vi "D2SParser - Private - Function - Read Character Stats.vi"(8 "error in (no error)":errorcluster, 11 "D2SParser in":refnum<class "D2SParser.lvclass">) -> (0 "error out":errorcluster, 3 "D2SParser out":refnum<class "D2SParser.lvclass">)   [LabVIEW 2015, in "D2SParser.lvclass"]
uses:
  D2SParser.lvclass
  D2SParser.lvclass/D2SParser.ctl
  D2Character/D2Character.lvclass/D2Character.ctl
  D2Character/D2Character - Accessors - Set Strength.vi
  D2Character/D2Character - Accessors - Set Energy.vi
  D2Character/D2Character - Accessors - Set Dexterity.vi
  D2Character/D2Character - Accessors - Set Vitality.vi
  D2Character/D2Character - Accessors - Set Stat Points Remaining.vi
  D2Character/D2Character - Accessors - Set Skill Points Remaining.vi
  D2Character/D2Character - Accessors - Set Current Life.vi
  D2Character/D2Character - Accessors - Set Life Base.vi
  D2Character/D2Character - Accessors - Set Current Mana.vi
  D2Character/D2Character - Accessors - Set Mana Base.vi
  D2Character/D2Character - Accessors - Set Current Stamina.vi
  D2Character/D2Character - Accessors - Set Stamina Base.vi
  D2Character/D2Character - Accessors - Set Level.vi
  D2Character/D2Character - Accessors - Set Experience.vi
  D2Character/D2Character - Accessors - Set Gold Inventory.vi
  D2Character/D2Character - Accessors - Set Stash Gold.vi
  D2Character/D2Character.lvclass
panel:
  out "ASCII":string
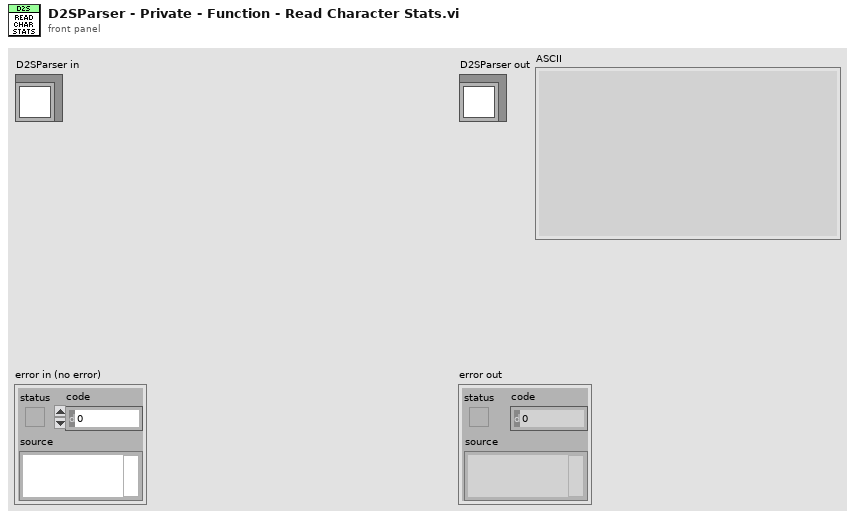
[diagram p1: front panel]
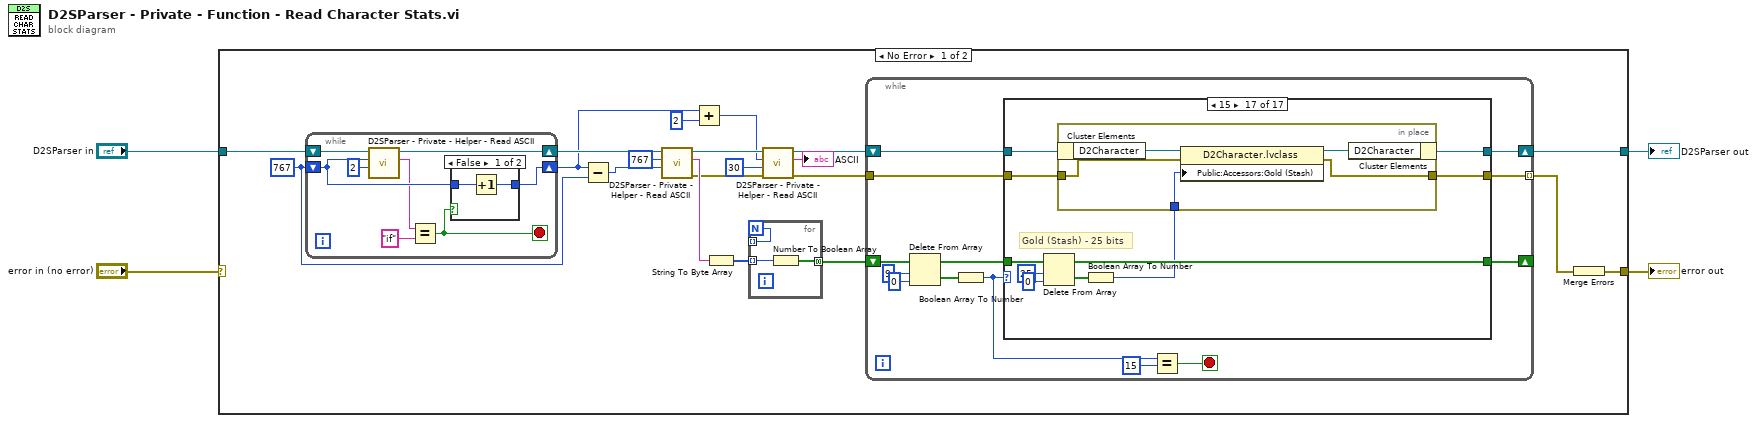
[diagram p0: block diagram]
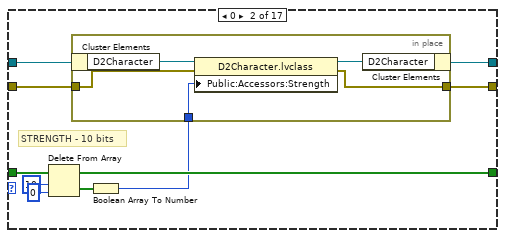
[diagram p3: hidden frame]
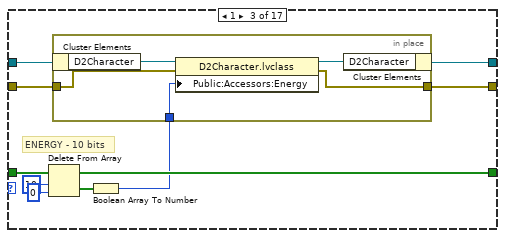
[diagram p4: hidden frame]
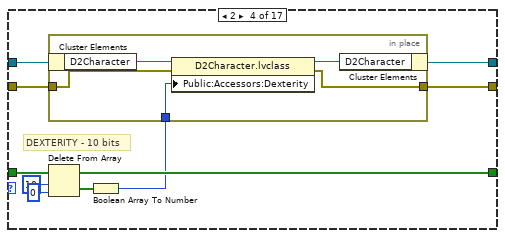
[diagram p5: hidden frame]
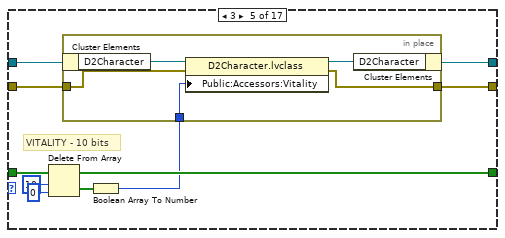
[diagram p6: hidden frame]
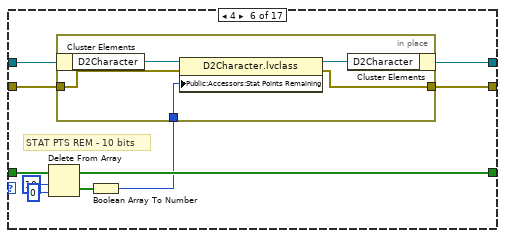
[diagram p7: hidden frame]
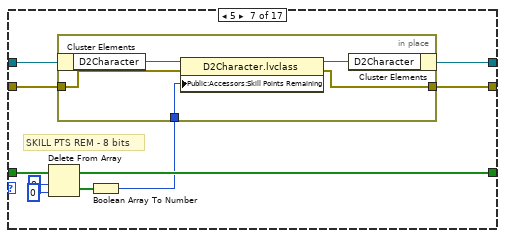
[diagram p8: hidden frame]
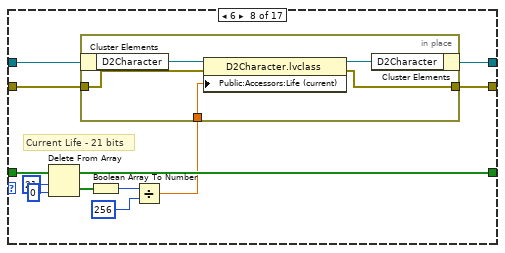
[diagram p9: hidden frame]
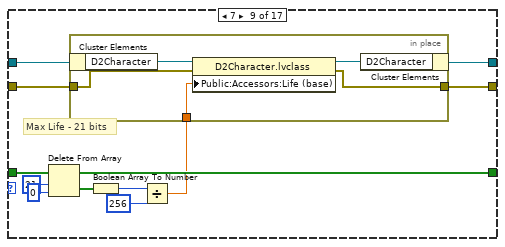
[diagram p10: hidden frame]
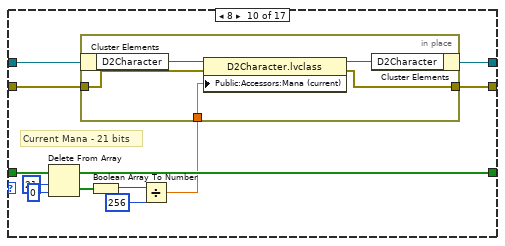
[diagram p11: hidden frame]
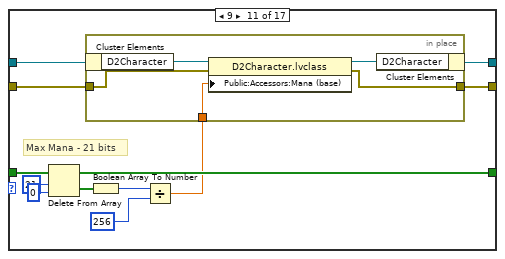
[diagram p12: hidden frame]
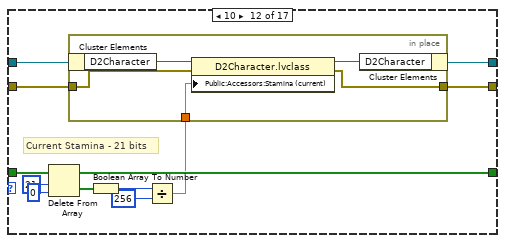
[diagram p13: hidden frame]
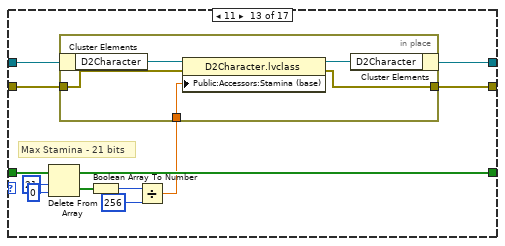
[diagram p14: hidden frame]
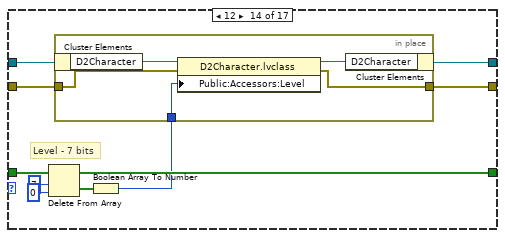
[diagram p15: hidden frame]
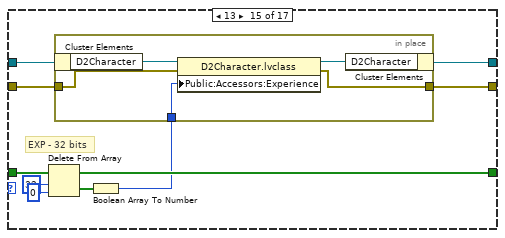
[diagram p16: hidden frame]
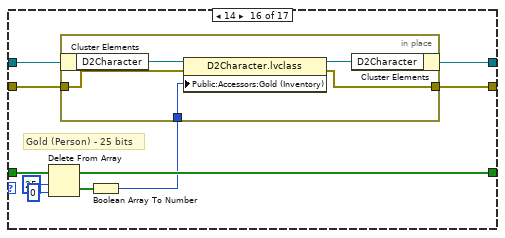
[diagram p17: hidden frame]
diagram:
  n1 = case shown="No Error" "error in (no error)" {
    selector: "error in (no error)" -> [_ w308]
    tunnel: [w22 w308] -> w3
    tunnel: [w23 w307] -> w1
    tunnel: "D2SParser in" -> [w24 w307]
    frame No Error {
      w21 = i64 767 ("Position")
      n2 = while {
        shift-right: [w301] -> w9
        shift-left: w21 -> [w302]
        shift-right: [w296] -> w20
        shift-left: w24 -> [w303]
        stop <- w297 stop-if-true
        n3 = call "D2SParser - Private - Helper - Read ASCII.vi"("# Characters"=2, "Position"=w302, "D2SParser in"=w303) -> ("ASCII"=w299:string, "D2SParser out"=w296:refnum<class "D2SParser.lvclass">)  [unwired: 6 in, 1 out]
        n4 = Equal?(x=w299, y="if") -> (x = y?=w297:bool)
        n5 = case shown="False" w297 {
          tunnel: w302 -> [w305 w306]
          tunnel: [w304 w306] -> w301
          frame False {
            n6 = Increment(x=w305) -> (x+1=w304:i64)
          }
          frame True {
          }
        }
      }
      n7 = Subtract(x=w9, y=w21) -> (x-y=w19:i64)
      n8 = call "D2SParser - Private - Helper - Read ASCII.vi"("# Characters"=w19, "Position"=i64 767, "D2SParser in"=w20) -> ("error out"=w11:errorcluster, "ASCII"=w17:string, "D2SParser out"=w13:refnum<class "D2SParser.lvclass">)  [unwired: 6 in]
      n9 = Add(x=w9, y=i64 2) -> (x+y=w8:i64)
      n10 = String To Byte Array(string=w17) -> (unsigned byte array=w16:u8[])
      n11 = for {
        N -> [w293]
        tunnel: w16 -> [w295] mode=indexing
        tunnel: [w294] -> w15 mode=concatenating
        tunnel: [w293] -> _ mode=indexing
        n12 = Number To Boolean Array(number=w295) -> (Boolean array=w294:bool[])
      }
      n13 = call "D2SParser - Private - Helper - Read ASCII.vi"("error in (no error)"=w11, "# Characters"=i64 30 ("x+y"), "Position"=w8, "D2SParser in"=w13) -> ("error out"=w10:errorcluster, "ASCII"=→"ASCII":string, "D2SParser out"=w12:refnum<class "D2SParser.lvclass">)  [unwired: 5 in]
      n14 = while {
        shift-right: [w32] -> _
        shift-left: w15 -> [w37]
        tunnel: w10 -> [w26]
        tunnel: [w25] -> w14 mode=indexing
        shift-right: [w27] -> w23
        shift-left: w12 -> [w28]
        stop <- w31 stop-if-true
        n15 = Delete From Array(array=w37, length=9, index=0) -> (deleted portion=w34:bool[], array with subset deleted=w33:bool[])
        n16 = Boolean Array To Number(Boolean array=w34) -> (number=w30:u32)
        n17 = case shown="15" w30 {
          tunnel: w33 -> [w40 w50 w65 w80 w95 w110 w125 w142 w159 w176 w193 w210 w227 w242 w257 w272 w287]
          tunnel: [w40 w47 w62 w77 w92 w107 w122 w139 w156 w173 w190 w207 w224 w239 w254 w269 w284] -> w32
          tunnel: w28 -> [w39 w45 w60 w75 w90 w105 w120 w133 w152 w171 w187 w205 w222 w237 w252 w267 w282]
          tunnel: [w39 w43 w57 w72 w88 w103 w118 w132 w149 w166 w186 w203 w220 w234 w249 w265 w279] -> w27
          tunnel: w26 -> [w38 w42 w58 w74 w89 w104 w119 w134 w151 w170 w188 w204 w221 w236 w251 w266 w281]
          tunnel: [w38 w44 w56 w71 w87 w102 w117 w135 w148 w165 w185 w202 w219 w233 w248 w264 w278] -> w25
          frame Default {
          }
          frame 0 {
            # "STRENGTH - 10 bits"
            n18 = Delete From Array(array=w50, length=10, index=0) -> (deleted portion=w46:bool[], array with subset deleted=w47:bool[])
            n19 = Boolean Array To Number(Boolean array=w46) -> (number=w41:u32)
            n20 = in-place {
              in-place-border: [w53] -> w44
              in-place-border: w42 -> [w52]
              in-place-border: w41 -> [w51]
              n21 = in-place-cluster #1(w45) -> ("D2Character"=w55:refnum<class "D2Character.lvclass">)
              n22 = property class="D2Character.lvclass"(reference=w55, error in=w52, "Public:Accessors:Strength"=w51) -> (reference out=w54:refnum<class "D2Character.lvclass">, error out=w53:errorcluster)
              n23 = in-place-cluster #1("D2Character"=w54) -> (w43:refnum<class "D2SParser.lvclass">)
            }
          }
          frame 1 {
            # "ENERGY - 10 bits"
            n24 = Delete From Array(array=w65, length=10, index=0) -> (deleted portion=w61:bool[], array with subset deleted=w62:bool[])
            n25 = Boolean Array To Number(Boolean array=w61) -> (number=w59:u32)
            n26 = in-place {
              in-place-border: [w68] -> w56
              in-place-border: w58 -> [w67]
              in-place-border: w59 -> [w66]
              n27 = in-place-cluster #2(w60) -> ("D2Character"=w70:refnum<class "D2Character.lvclass">)
              n28 = property class="D2Character.lvclass"(reference=w70, error in=w67, "Public:Accessors:Energy"=w66) -> (reference out=w69:refnum<class "D2Character.lvclass">, error out=w68:errorcluster)
              n29 = in-place-cluster #2("D2Character"=w69) -> (w57:refnum<class "D2SParser.lvclass">)
            }
          }
          frame 2 {
            # "DEXTERITY - 10 bits"
            n30 = Delete From Array(array=w80, length=10, index=0) -> (deleted portion=w76:bool[], array with subset deleted=w77:bool[])
            n31 = Boolean Array To Number(Boolean array=w76) -> (number=w73:u32)
            n32 = in-place {
              in-place-border: [w83] -> w71
              in-place-border: w74 -> [w82]
              in-place-border: w73 -> [w81]
              n33 = in-place-cluster #3(w75) -> ("D2Character"=w85:refnum<class "D2Character.lvclass">)
              n34 = property class="D2Character.lvclass"(reference=w85, error in=w82, "Public:Accessors:Dexterity"=w81) -> (reference out=w84:refnum<class "D2Character.lvclass">, error out=w83:errorcluster)
              n35 = in-place-cluster #3("D2Character"=w84) -> (w72:refnum<class "D2SParser.lvclass">)
            }
          }
          frame 3 {
            # "VITALITY - 10 bits"
            n36 = Delete From Array(array=w95, length=10, index=0) -> (deleted portion=w91:bool[], array with subset deleted=w92:bool[])
            n37 = Boolean Array To Number(Boolean array=w91) -> (number=w86:u32)
            n38 = in-place {
              in-place-border: [w98] -> w87
              in-place-border: w89 -> [w97]
              in-place-border: w86 -> [w96]
              n39 = in-place-cluster #4(w90) -> ("D2Character"=w100:refnum<class "D2Character.lvclass">)
              n40 = property class="D2Character.lvclass"(reference=w100, error in=w97, "Public:Accessors:Vitality"=w96) -> (reference out=w99:refnum<class "D2Character.lvclass">, error out=w98:errorcluster)
              n41 = in-place-cluster #4("D2Character"=w99) -> (w88:refnum<class "D2SParser.lvclass">)
            }
          }
          frame 4 {
            # "STAT PTS REM - 10 bits"
            n42 = Delete From Array(array=w110, length=10, index=0) -> (deleted portion=w106:bool[], array with subset deleted=w107:bool[])
            n43 = Boolean Array To Number(Boolean array=w106) -> (number=w101:u32)
            n44 = in-place {
              in-place-border: [w113] -> w102
              in-place-border: w104 -> [w112]
              in-place-border: w101 -> [w111]
              n45 = in-place-cluster #5(w105) -> ("D2Character"=w115:refnum<class "D2Character.lvclass">)
              n46 = property class="D2Character.lvclass"(reference=w115, error in=w112, "Public:Accessors:Stat Points Remaining"=w111) -> (reference out=w114:refnum<class "D2Character.lvclass">, error out=w113:errorcluster)
              n47 = in-place-cluster #5("D2Character"=w114) -> (w103:refnum<class "D2SParser.lvclass">)
            }
          }
          frame 5 {
            # "SKILL PTS REM - 8 bits"
            n48 = Delete From Array(array=w125, length=8, index=0) -> (deleted portion=w121:bool[], array with subset deleted=w122:bool[])
            n49 = Boolean Array To Number(Boolean array=w121) -> (number=w116:u32)
            n50 = in-place {
              in-place-border: [w128] -> w117
              in-place-border: w119 -> [w127]
              in-place-border: w116 -> [w126]
              n51 = in-place-cluster #6(w120) -> ("D2Character"=w130:refnum<class "D2Character.lvclass">)
              n52 = property class="D2Character.lvclass"(reference=w130, error in=w127, "Public:Accessors:Skill Points Remaining"=w126) -> (reference out=w129:refnum<class "D2Character.lvclass">, error out=w128:errorcluster)
              n53 = in-place-cluster #6("D2Character"=w129) -> (w118:refnum<class "D2SParser.lvclass">)
            }
          }
          frame 6 {
            # "Current Life - 21 bits"
            n54 = Delete From Array(array=w142, length=21, index=0) -> (deleted portion=w138:bool[], array with subset deleted=w139:bool[])
            n55 = Boolean Array To Number(Boolean array=w138) -> (number=w137:u32)
            n56 = Divide(x=w137, y=u32 256) -> (x/y=w131:dbl)
            n57 = in-place {
              in-place-border: [w146] -> w135
              in-place-border: w134 -> [w145]
              in-place-border: w131 -> [w144]
              n58 = in-place-cluster #7(w133) -> ("D2Character"=w143:refnum<class "D2Character.lvclass">)
              n59 = property class="D2Character.lvclass"(reference=w143, error in=w145, "Public:Accessors:Life (current)"=w144) -> (reference out=w147:refnum<class "D2Character.lvclass">, error out=w146:errorcluster)
              n60 = in-place-cluster #7("D2Character"=w147) -> (w132:refnum<class "D2SParser.lvclass">)
            }
          }
          frame 7 {
            # "Max Life - 21 bits"
            n61 = Delete From Array(array=w159, length=21, index=0) -> (deleted portion=w155:bool[], array with subset deleted=w156:bool[])
            n62 = Boolean Array To Number(Boolean array=w155) -> (number=w154:u32)
            n63 = Divide(x=w154, y=u32 256) -> (x/y=w150:dbl)
            n64 = in-place {
              in-place-border: [w162] -> w148
              in-place-border: w151 -> [w161]
              in-place-border: w150 -> [w160]
              n65 = in-place-cluster #8(w152) -> ("D2Character"=w164:refnum<class "D2Character.lvclass">)
              n66 = property class="D2Character.lvclass"(reference=w164, error in=w161, "Public:Accessors:Life (base)"=w160) -> (reference out=w163:refnum<class "D2Character.lvclass">, error out=w162:errorcluster)
              n67 = in-place-cluster #8("D2Character"=w163) -> (w149:refnum<class "D2SParser.lvclass">)
            }
          }
          frame 8 {
            # "Current Mana - 21 bits"
            n68 = Delete From Array(array=w176, length=21, index=0) -> (deleted portion=w172:bool[], array with subset deleted=w173:bool[])
            n69 = Boolean Array To Number(Boolean array=w172) -> (number=w169:u32)
            n70 = Divide(x=w169, y=u32 256) -> (x/y=w167:dbl)
            n71 = in-place {
              in-place-border: [w179] -> w165
              in-place-border: w170 -> [w178]
              in-place-border: w167 -> [w177]
              n72 = in-place-cluster #9(w171) -> ("D2Character"=w181:refnum<class "D2Character.lvclass">)
              n73 = property class="D2Character.lvclass"(reference=w181, error in=w178, "Public:Accessors:Mana (current)"=w177) -> (reference out=w180:refnum<class "D2Character.lvclass">, error out=w179:errorcluster)
              n74 = in-place-cluster #9("D2Character"=w180) -> (w166:refnum<class "D2SParser.lvclass">)
            }
          }
          frame 9 {
            # "Max Mana - 21 bits"
            n75 = Delete From Array(array=w193, length=21, index=0) -> (deleted portion=w189:bool[], array with subset deleted=w190:bool[])
            n76 = Boolean Array To Number(Boolean array=w189) -> (number=w184:u32)
            n77 = Divide(x=w184, y=u32 256) -> (x/y=w183:dbl)
            n78 = in-place {
              in-place-border: [w196] -> w185
              in-place-border: w188 -> [w195]
              in-place-border: w183 -> [w194]
              n79 = in-place-cluster #10(w187) -> ("D2Character"=w198:refnum<class "D2Character.lvclass">)
              n80 = property class="D2Character.lvclass"(reference=w198, error in=w195, "Public:Accessors:Mana (base)"=w194) -> (reference out=w197:refnum<class "D2Character.lvclass">, error out=w196:errorcluster)
              n81 = in-place-cluster #10("D2Character"=w197) -> (w186:refnum<class "D2SParser.lvclass">)
            }
          }
          frame 10 {
            # "Current Stamina - 21 bits"
            n82 = Delete From Array(array=w210, length=21, index=0) -> (deleted portion=w206:bool[], array with subset deleted=w207:bool[])
            n83 = Boolean Array To Number(Boolean array=w206) -> (number=w201:u32)
            n84 = Divide(x=w201, y=u32 256) -> (x/y=w199:dbl)
            n85 = in-place {
              in-place-border: [w213] -> w202
              in-place-border: w204 -> [w212]
              in-place-border: w199 -> [w211]
              n86 = in-place-cluster #11(w205) -> ("D2Character"=w215:refnum<class "D2Character.lvclass">)
              n87 = property class="D2Character.lvclass"(reference=w215, error in=w212, "Public:Accessors:Stamina (current)"=w211) -> (reference out=w214:refnum<class "D2Character.lvclass">, error out=w213:errorcluster)
              n88 = in-place-cluster #11("D2Character"=w214) -> (w203:refnum<class "D2SParser.lvclass">)
            }
          }
          frame 11 {
            # "Max Stamina - 21 bits"
            n89 = Delete From Array(array=w227, length=21, index=0) -> (deleted portion=w223:bool[], array with subset deleted=w224:bool[])
            n90 = Boolean Array To Number(Boolean array=w223) -> (number=w218:u32)
            n91 = Divide(x=w218, y=u32 256) -> (x/y=w216:dbl)
            n92 = in-place {
              in-place-border: [w230] -> w219
              in-place-border: w221 -> [w229]
              in-place-border: w216 -> [w228]
              n93 = in-place-cluster #12(w222) -> ("D2Character"=w232:refnum<class "D2Character.lvclass">)
              n94 = property class="D2Character.lvclass"(reference=w232, error in=w229, "Public:Accessors:Stamina (base)"=w228) -> (reference out=w231:refnum<class "D2Character.lvclass">, error out=w230:errorcluster)
              n95 = in-place-cluster #12("D2Character"=w231) -> (w220:refnum<class "D2SParser.lvclass">)
            }
          }
          frame 12 {
            # "Level - 7 bits"
            n96 = Delete From Array(array=w242, length=7, index=0) -> (deleted portion=w238:bool[], array with subset deleted=w239:bool[])
            n97 = Boolean Array To Number(Boolean array=w238) -> (number=w235:u32)
            n98 = in-place {
              in-place-border: [w245] -> w233
              in-place-border: w236 -> [w244]
              in-place-border: w235 -> [w243]
              n99 = in-place-cluster #13(w237) -> ("D2Character"=w247:refnum<class "D2Character.lvclass">)
              n100 = property class="D2Character.lvclass"(reference=w247, error in=w244, "Public:Accessors:Level"=w243) -> (reference out=w246:refnum<class "D2Character.lvclass">, error out=w245:errorcluster)
              n101 = in-place-cluster #13("D2Character"=w246) -> (w234:refnum<class "D2SParser.lvclass">)
            }
          }
          frame 13 {
            # "EXP - 32 bits"
            n102 = Delete From Array(array=w257, length=32, index=0) -> (deleted portion=w253:bool[], array with subset deleted=w254:bool[])
            n103 = Boolean Array To Number(Boolean array=w253) -> (number=w250:u32)
            n104 = in-place {
              in-place-border: [w260] -> w248
              in-place-border: w251 -> [w259]
              in-place-border: w250 -> [w258]
              n105 = in-place-cluster #14(w252) -> ("D2Character"=w262:refnum<class "D2Character.lvclass">)
              n106 = property class="D2Character.lvclass"(reference=w262, error in=w259, "Public:Accessors:Experience"=w258) -> (reference out=w261:refnum<class "D2Character.lvclass">, error out=w260:errorcluster)
              n107 = in-place-cluster #14("D2Character"=w261) -> (w249:refnum<class "D2SParser.lvclass">)
            }
          }
          frame 14 {
            # "Gold (Person) - 25 bits"
            n108 = Delete From Array(array=w272, length=25, index=0) -> (deleted portion=w268:bool[], array with subset deleted=w269:bool[])
            n109 = Boolean Array To Number(Boolean array=w268) -> (number=w263:u32)
            n110 = in-place {
              in-place-border: [w275] -> w264
              in-place-border: w266 -> [w274]
              in-place-border: w263 -> [w273]
              n111 = in-place-cluster #15(w267) -> ("D2Character"=w277:refnum<class "D2Character.lvclass">)
              n112 = property class="D2Character.lvclass"(reference=w277, error in=w274, "Public:Accessors:Gold (Inventory)"=w273) -> (reference out=w276:refnum<class "D2Character.lvclass">, error out=w275:errorcluster)
              n113 = in-place-cluster #15("D2Character"=w276) -> (w265:refnum<class "D2SParser.lvclass">)
            }
          }
          frame 15 {
            # "Gold (Stash) - 25 bits"
            n114 = Delete From Array(array=w287, length=25, index=0) -> (deleted portion=w283:bool[], array with subset deleted=w284:bool[])
            n115 = Boolean Array To Number(Boolean array=w283) -> (number=w280:u32)
            n116 = in-place {
              in-place-border: [w290] -> w278
              in-place-border: w281 -> [w289]
              in-place-border: w280 -> [w288]
              n117 = in-place-cluster #16(w282) -> ("D2Character"=w292:refnum<class "D2Character.lvclass">)
              n118 = property class="D2Character.lvclass"(reference=w292, error in=w289, "Public:Accessors:Gold (Stash)"=w288) -> (reference out=w291:refnum<class "D2Character.lvclass">, error out=w290:errorcluster)
              n119 = in-place-cluster #16("D2Character"=w291) -> (w279:refnum<class "D2SParser.lvclass">)
            }
          }
        }
        n120 = Equal?(x=w30, y=u32 15) -> (x = y?=w31:bool)
      }
      n121 = Merge Errors(w14) -> (w22:errorcluster)
    }
    frame Error {
    }
  }
  "error out" <- w3
  "D2SParser out" <- w1
